vi "GE 5565PIORC.PXI Interrupts.Enable.vi"(8 "error in (no error)":errorcluster, 10 "Enable Interrupts":bool=TRUE, 11 "GE 5565PIORC in":refnum<class "GE 5565PIORC.lvclass">) -> (0 "error out":errorcluster, 3 "GE 5565PIORC out":refnum<class "GE 5565PIORC.lvclass">)   [LabVIEW 2016, in "GE 5565PIORC.lvclass"]
doc: "Enable or disable PXI Interrupts for the GE 5565PIORC. Interrupts are required for certain aspects of DMA transfers to function correctly."
uses:
  GE 5565PIORC.lvclass
  GE 5565PIORC.lvclass/GE 5565PIORC.ctl
  <vilib>/Instr/_visa.llb/Select Event Type.ctl
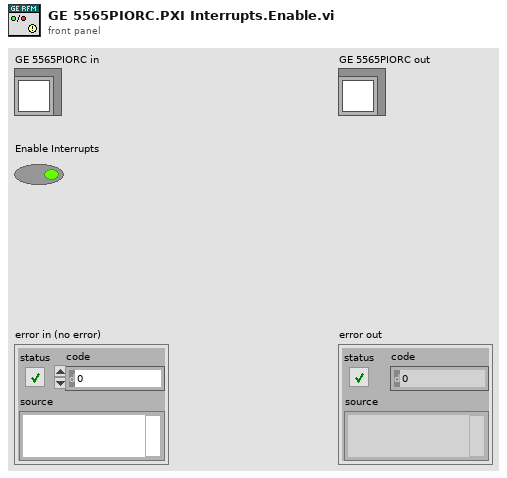
[diagram p1: front panel]
types:
  T1 = typedef "Select Event Type.ctl" = u32
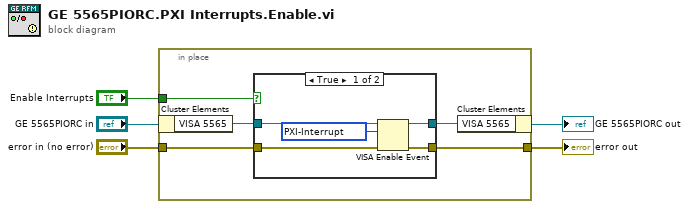
[diagram p0: block diagram]
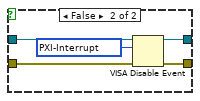
[diagram p2: hidden frame]
diagram:
  n1 = in-place {
    in-place-border: "error in (no error)" -> [w9]
    in-place-border: [w8] -> w3
    in-place-border: "Enable Interrupts" -> [w6]
    n2 = in-place-cluster #1("GE 5565PIORC in") -> ("VISA 5565"=w10:refnum<visa-resource-name>)
    n3 = case shown="True" w6 {
      tunnel: w10 -> [w14 w19]
      tunnel: w9 -> [w13 w18]
      tunnel: [w12 w17] -> w8
      tunnel: [w11 w16] -> w7
      frame True {
        w15 = T1 1073684514 items=["ServiceRequest"=1073684491, "Trigger"=3221168138, "Clear"=1073684493, "VXI-Signal"=1073684512, "VXI/VME-Interrupt"=3221168161, "VXI/VME-Sysfail"=1073684509, "VXI/VME-Sysreset"=1073684510, "GPIB-CIC"=1073684498, "GPIB-Talk"=1073684499, "GPIB-Listen"=1073684500, "PXI-Interrupt"=1073684514, "AllEnabled"=1073709055] ("Event Type")
        n4 = VISA Enable Event(8:w13, 10:w15, 11:w14) -> (0:w12:errorcluster, 3:w11:refnum<visa-resource-name>)  [unwired: 1 in]
      }
      frame False {
        w20 = T1 1073684514 items=["ServiceRequest"=1073684491, "Trigger"=3221168138, "Clear"=1073684493, "VXI-Signal"=1073684512, "VXI/VME-Interrupt"=3221168161, "VXI/VME-Sysfail"=1073684509, "VXI/VME-Sysreset"=1073684510, "GPIB-CIC"=1073684498, "GPIB-Talk"=1073684499, "GPIB-Listen"=1073684500, "PXI-Interrupt"=1073684514, "AllEnabled"=1073709055] ("Event Type")
        n5 = VISA Disable Event(8:w18, 10:w20, 11:w19) -> (0:w17:errorcluster, 3:w16:refnum<visa-resource-name>)  [unwired: 1 in]
      }
    }
    n6 = in-place-cluster #1("VISA 5565"=w7) -> (→"GE 5565PIORC out":refnum<class "GE 5565PIORC.lvclass">)
  }
  "error out" <- w3
